vi "Parse Close Delimiter.vi"(8 "Error In":errorcluster, 11 "Parser In":refnum<class "Lexer.lvclass">) -> (0 "Error Out":errorcluster, 3 "Parser Out":refnum<class "Lexer.lvclass">)   [LabVIEW 2018, in "Toolkit.lvlib" / "Lexer.lvclass"]
uses:
  Lexer.lvclass
  Lexer.lvclass/Lexer.ctl
  Type Definitions/States.ctl
  Tokens/EscapedVariable/EscapedVariable.lvclass
  D:/Users/cfield/Code/Field R&D Services/Mustache/trunk/src/Toolkit/Tokens/Keyable/API/Keyable.lvclass
  Tokens/UnescapedVariable/UnescapedVariable.lvclass
  Tokens/BeginSection/BeginSection.lvclass
  Tokens/InvertedSection/InvertedSection.lvclass
  Tokens/EndSection/EndSection.lvclass
  Tokens/Partial/Partial.lvclass
  Tokens/Keyable/API/Keyable.lvclass
  D:/Users/cfield/Code/Field R&D Services/Mustache/trunk/src/Toolkit/Tokens/Abstract/Abstract.lvclass
  <vilib>/Utility/error.llb/Trim Whitespace.vi
  Tokens/EscapedVariable/API/New.vi
  Tokens/UnescapedVariable/API/New.vi
  Tokens/BeginSection/API/New.vi
  Tokens/InvertedSection/API/New.vi
  Tokens/EndSection/API/New.vi
  Tokens/Partial/API/New.vi
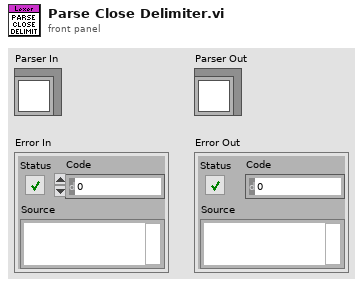
[diagram p1: front panel]
types:
  T1 = typedef "Toolkit.lvlib/Lexer.lvclass/States.ctl" = enum16{"Text", "Open Delimiter", "Tag Type", "Tag Key", "Close Delimiter"}
  T2 = typedef "Toolkit.lvlib/Lexer.lvclass/Tag Types.ctl" = enum16{"Escaped Variable", "{} Unescaped Variable", "& Unescaped Variable", "Begin Section", "Inverted Section", "End Section", "Comment", "Partial", "Set Delimiter"}
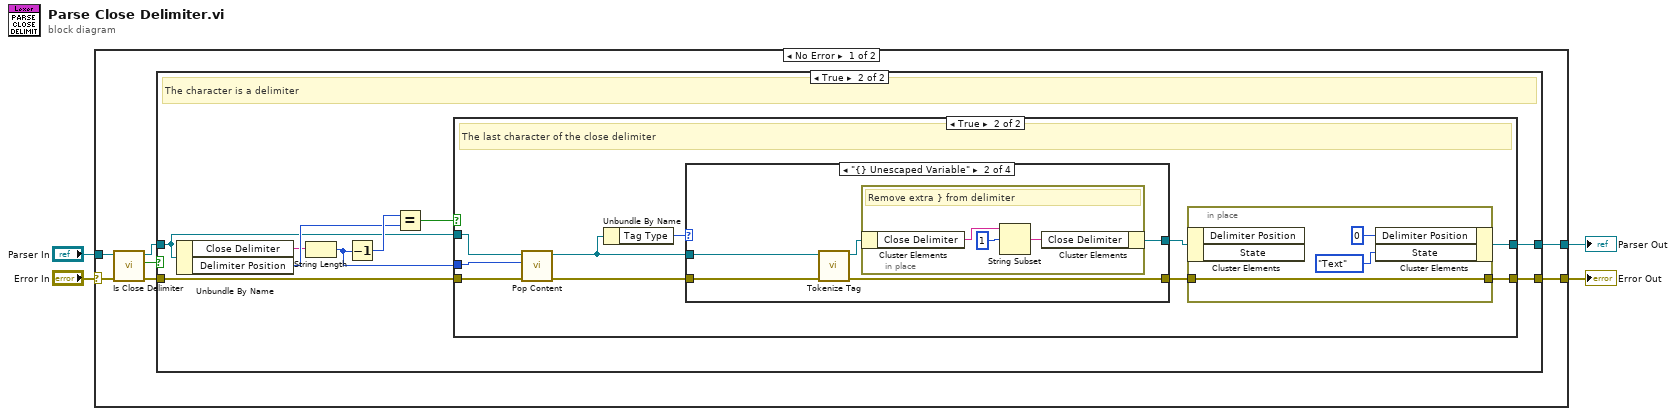
[diagram p0: block diagram]
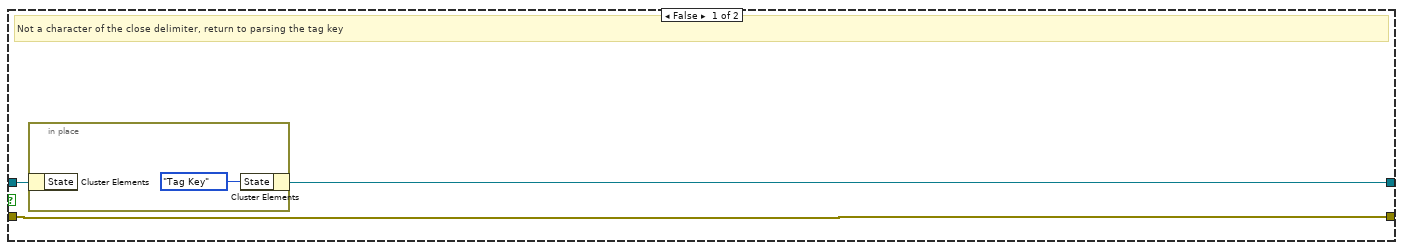
[diagram p2: hidden frame]
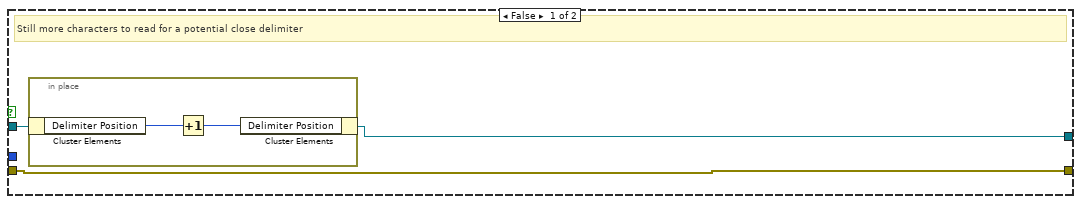
[diagram p3: hidden frame]
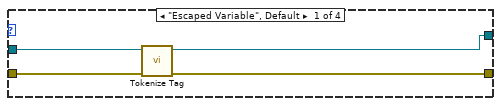
[diagram p4: hidden frame]
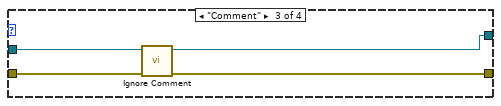
[diagram p5: hidden frame]
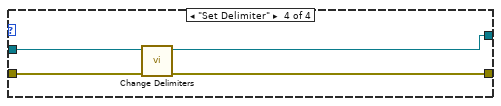
[diagram p6: hidden frame]
diagram:
  n1 = case shown="No Error" "Error In" {
    selector: "Error In" -> [w10 w63]
    tunnel: [w6 w63] -> w4
    tunnel: [w5 w64] -> w3
    tunnel: "Parser In" -> [w11 w64]
    frame No Error {
      n2 = call "Is Close Delimiter.vi"("Error In"=w10, "Parser In"=w11) -> ("Error Out"=w9:errorcluster, "Close Delimiter"=w7:bool, "Parser Out"=w8:refnum<class "Lexer.lvclass">)  [unwired: 7 in]
      n3 = case shown="True" w7 {
        tunnel: w9 -> [w14 w21]
        tunnel: w8 -> [w13 w20]
        tunnel: [w14 w18] -> w6
        tunnel: [w12 w19] -> w5
        frame False {
          # "Not a character of the close delimiter, return to parsing the tag key"
          n4 = in-place {
            n5 = in-place-cluster #1(w13) -> ()  [unwired: 1 out]
            n6 = in-place-cluster #1("State"=States."Tag Key") -> (w12:refnum<class "Lexer.lvclass">)
          }
        }
        frame True {
          # "The character is a delimiter"
          n7 = Unbundle By Name(w20) -> ("Close Delimiter"=w17:string, "Delimiter Position"=w23:i32)
          n8 = String Length(string=w17) -> (length=w16:i32)
          n9 = Decrement(x=w16) -> (x-1=w24:i32)
          n10 = Equal?(x=w24, y=w23) -> (x = y?=w22:bool)
          n11 = case shown="True" w22 {
            tunnel: w21 -> [w25 w39]
            tunnel: w20 -> [w27 w35]
            tunnel: [w26 w32] -> w19
            tunnel: [w25 w36] -> w18
            tunnel: w16 -> [_ w33]
            frame False {
              # "Still more characters to read for a potential close delimiter"
              n12 = in-place {
                n13 = in-place-cluster #2(w27) -> ("Delimiter Position"=w29:i32)
                n14 = Increment(x=w29) -> (x+1=w28:i32)
                n15 = in-place-cluster #2("Delimiter Position"=w28) -> (w26:refnum<class "Lexer.lvclass">)
              }
            }
            frame True {
              # "The last character of the close delimiter"
              n16 = call "Pop Content.vi"("Error In"=w39, "Characters Count"=w33, "Parser In"=w35) -> ("Error Out"=w34:errorcluster, "Parser Out"=w31:refnum<class "Lexer.lvclass">)  [unwired: 7 in]
              n17 = Unbundle By Name(w31) -> ("Tag Type"=w30:T2)
              n18 = case shown="\"{} Unescaped Variable\"" w30 {
                tunnel: [w43 w44 w54 w57] -> w38
                tunnel: [w42 w48 w53 w56] -> w37
                tunnel: w34 -> [w41 w47 w52 w58]
                tunnel: w31 -> [w40 w46 w55 w59]
                frame "Escaped Variable", Default {
                  n19 = call "Tokenize Tag.vi"("Error In"=w41, "Parser In"=w40) -> ("Error Out"=w42:errorcluster, "Parser Out"=w43:refnum<class "Lexer.lvclass">)  [unwired: 8 in]
                }
                frame "{} Unescaped Variable" {
                  n20 = call "Tokenize Tag.vi"("Error In"=w47, "Parser In"=w46) -> ("Error Out"=w48:errorcluster, "Parser Out"=w45:refnum<class "Lexer.lvclass">)  [unwired: 8 in]
                  n21 = in-place {
                    # "Remove extra } from delimiter"
                    n22 = in-place-cluster #3(w45) -> ("Close Delimiter"=w51:string)
                    n23 = String Subset(string=w51, offset (0)=1) -> (substring=w49:string)  [unwired: 1 in]
                    n24 = in-place-cluster #3("Close Delimiter"=w49) -> (w44:refnum<class "Lexer.lvclass">)
                  }
                }
                frame "Comment" {
                  n25 = call "Ignore Comment.vi"("Error In"=w52, "Parser In"=w55) -> ("Error Out"=w53:errorcluster, "Parser Out"=w54:refnum<class "Lexer.lvclass">)  [unwired: 8 in]
                }
                frame "Set Delimiter" {
                  n26 = call "Change Delimiters.vi"("Error In"=w58, "Parser In"=w59) -> ("Error Out"=w56:errorcluster, "Parser Out"=w57:refnum<class "Lexer.lvclass">)  [unwired: 8 in]
                }
              }
              n27 = in-place {
                in-place-border: w37 -> [w62]
                in-place-border: [w62] -> w36
                n28 = in-place-cluster #4(w38) -> ()  [unwired: 2 out]
                n29 = in-place-cluster #4("Delimiter Position"=0, "State"=States."Text") -> (w32:refnum<class "Lexer.lvclass">)
              }
            }
          }
        }
      }
    }
    frame Error {
    }
  }
  "Error Out" <- w4
  "Parser Out" <- w3
